vi "MainIdent RT.vi"() -> ()   [LabVIEW 2019]
doc: "The myRIO Project template acquires acceleration data from the onboard accelerometer and displays the changes of acceleration values in a waveform chart."
uses:
  <vilib>/myRIO/Common/Instrument Driver Framework/myRIO v1.0/Encoder/typedefs/Encoder Signal Mode.ctl
  <vilib>/Platform/TimedLoop/XDataNode/timing_clust.ctl
  <vilib>/Platform/TimedLoop/XDataNode/nitl_modes.ctl
  <vilib>/Platform/TimedLoop/XDataNode/wakeup.ctl
  <vilib>/myRIO/Instrument Drivers/Onboard IO/PWM/typedefs/PWM Reference.ctl
  <vilib>/myRIO/Common/Instrument Driver Framework/Utilities/typedefs/myRIO Generic Hardware Reference.ctl
  <vilib>/myRIO/Common/Instrument Driver Framework/Utilities/typedefs/Hardware Version Enum.ctl
  <vilib>/myRIO/Common/Instrument Driver Framework/Utilities/typedefs/myRIO v1.0 Reference.ctl
  <vilib>/myRIO/Common/Instrument Driver Framework/Utilities/typedefs/Generic FPGA Reference.ctl
  <vilib>/myRIO/Common/Instrument Driver Framework/myRIO v1.0/PWM/typedefs/PWM Channels Enum.ctl
  <vilib>/myRIO/Instrument Drivers/Onboard IO/PWM/typedefs/PWM Configuration.ctl
  <vilib>/userDefined/High Color/nirio_resource_hc.ctl
  <vilib>/myRIO/Common/Instrument Driver Framework/myRIO v1.0/Encoder/typedefs/Encoder Configuration v1.0.ctl
  <vilib>/myRIO/Instrument Drivers/Onboard IO/Encoder/typedefs/Encoder Reference.ctl
  <vilib>/myRIO/Common/Instrument Driver Framework/myRIO v1.0/Encoder/typedefs/Encoder Channels Enum.ctl
  <vilib>/myRIO/Common/Instrument Driver Framework/myRIO v1.0/PWM/vis/myRIO v1.1 Open PWM.vi
  <vilib>/myRIO/Common/Instrument Driver Framework/myRIO v1.0/Encoder/vis/myRIO v1.1 Open Encoder.vi
  <vilib>/myRIO/Common/Instrument Driver Framework/Utilities/vis/Validate Channels.vi
  <vilib>/myRIO/Common/Instrument Driver Framework/myRIO v1.0/PWM/vis/myRIO v1.0 Reserve PWM.vi
  <vilib>/myRIO/Instrument Drivers/Onboard IO/PWM/vis/Set Duty Cycle and Frequency.vi
  <vilib>/myRIO/Common/Instrument Driver Framework/myRIO v1.0/Encoder/vis/myRIO v1.0 Reserve Encoder.vi
  <vilib>/myRIO/Common/Instrument Driver Framework/myRIO v1.0/Encoder/vis/myRIO v1.0 Close Encoder.vi
  <vilib>/myRIO/Common/Instrument Driver Framework/myRIO v1.0/PWM/vis/myRIO v1.0 Close PWM.vi
  <vilib>/myRIO/Common/Instrument Driver Framework/myRIO v1.0/DIO/vis/myRIO v1.0 Close DIO.vi
  <vilib>/myRIO/Common/Instrument Driver Framework/myRIO v1.0/PWM/vis/myRIO v1.0 Build MUX Configuration PWM.vi
  <vilib>/myRIO/Common/Instrument Driver Framework/myRIO v1.0/Resource Manager/vis/myRIO v1.0 Reserve Channel List.vi
  <vilib>/myRIO/Common/Instrument Driver Framework/myRIO v1.0/Encoder/vis/myRIO v1.0 Build MUX Configuration Encoder.vi
  <vilib>/myRIO/Common/Instrument Driver Framework/myRIO v1.0/Encoder/vis/myRIO v1.0 Unreserve Encoder.vi
  <vilib>/myRIO/Common/Instrument Driver Framework/myRIO v1.0/PWM/vis/myRIO v1.0 Unreserve PWM.vi
  <vilib>/myRIO/Common/Instrument Driver Framework/myRIO v1.0/DIO/vis/myRIO v1.0 Unreserve DIO.vi
  <vilib>/myRIO/Common/Instrument Driver Framework/myRIO v1.0/Resource Manager/vis/myRIO v1.0 Create Configuration List.vi
  <vilib>/myRIO/Common/Instrument Driver Framework/myRIO v1.0/Resource Manager/vis/myRIO v1.0 Reserve Channel.vi
  <vilib>/myRIO/Common/Instrument Driver Framework/myRIO v1.0/Resource Manager/vis/myRIO v1.0 Unreserve Channel.vi
  <vilib>/myRIO/Common/Instrument Driver Framework/myRIO v1.0/Resource Manager/vis/myRIO v1.0 Unreserve Channel List.vi
  <vilib>/myRIO/Common/Instrument Driver Framework/myRIO v1.0/DIO/vis/myRIO v1.0 Build MUX Configuration DIO.vi
  <vilib>/myRIO/Common/Instrument Driver Framework/myRIO v1.0/Resource Manager/vis/myRIO v1.0 Build Mutex Name.vi
  <vilib>/Utility/VariantDataType/GetNumericInfo.vi
  <vilib>/Utility/error.llb/Error Cluster From Error Code.vi
  <vilib>/myRIO/Common/Instrument Driver Framework/myRIO v1.0/myRIO v1.1 Open.vi
  <vilib>/myRIO/Common/Instrument Driver Framework/Utilities/vis/IO Manager.vi
  <vilib>/myRIO/Common/Instrument Driver Framework/Utilities/vis/Configuration Manager.vi
  <vilib>/myRIO/Common/Instrument Driver Framework/myRIO v1.0/Resource Manager/vis/myRIO v1.0 Configure IO.vi
  <vilib>/myRIO/Common/Instrument Driver Framework/myRIO v1.0/myRIO v1.0 Close.vi
  <vilib>/myRIO/Common/Instrument Driver Framework/myRIO v1.0/PWM/vis/myRIO v1.0 Write PWM.vi
  <vilib>/myRIO/Common/Instrument Driver Framework/myRIO v1.0/Encoder/vis/myRIO v1.0 Configure Encoder.vi
  <vilib>/myRIO/Common/Instrument Driver Framework/myRIO v1.0/Encoder/vis/myRIO v1.0 Enable Encoder.vi
  <vilib>/myRIO/Common/Instrument Driver Framework/myRIO v1.0/Encoder/vis/myRIO v1.0 Read Encoder.vi
  <vilib>/myRIO/Common/Instrument Driver Framework/myRIO v1.0/Encoder/vis/myRIO v1.0 Shutdown Encoder.vi
  <vilib>/myRIO/Common/Instrument Driver Framework/myRIO v1.0/PWM/vis/myRIO v1.0 Shutdown PWM.vi
  <vilib>/myRIO/Common/Instrument Driver Framework/myRIO v1.0/DIO/vis/myRIO v1.0 Shutdown DIO.vi
  <vilib>/Platform/TimedLoop/XDataNode/XDataNode.xnode
  <vilib>/myRIO/Instrument Drivers/Onboard IO/PWM/vis/myRIO PWM Open.xnode
  <vilib>/myRIO/Instrument Drivers/Onboard IO/Encoder/vis/myRIO Encoder Open.xnode
  <vilib>/Platform/TimedLoop/XDataNode/XDNodeRunTimeDep.lvlib
  <vilib>/myRIO/Instrument Drivers/Onboard IO/Encoder/Encoder.lvlib
  <vilib>/myRIO/Instrument Drivers/Onboard IO/PWM/PWM.lvlib
  <vilib>/myRIO/Instrument Drivers/Onboard IO/DIO/DIO.lvlib
panel:
  in  "Reset Counter":bool
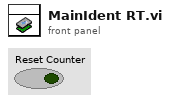
[diagram p1: front panel]
types:
  T1 = typedef "Encoder Signal Mode.ctl" = enum16{"Quadrature phase signal", "Step and direction signal"}
  T2 = typedef "PWM.lvlib/PWM Reference.ctl" = cluster{"myRIO Reference":T3, "PWM Channels Enum":T7, "PWM Configuration":T8}
  T3 = typedef "myRIO Generic Hardware Reference.ctl" = cluster{"myRIO Model":T4, "myRIO Hardware Reference":T5}
  T4 = typedef "Hardware Version Enum.ctl" = enum16{"Unknown", "myRIO-1900", "myRIO-1950", "roboRIO", "NI ELVIS RIO CM", "ELVIS III"}
  T5 = typedef "myRIO v1.0 Reference.ctl" = cluster{"Generic FPGA Reference":T6, "Allow multiple opens":bool}
  T6 = typedef "Generic FPGA Reference.ctl" = refnum<k20>
  T7 = typedef "PWM Channels Enum.ctl" = enum16{"Not Connected", "C/PWM0", "C/PWM1", "A/PWM0", "A/PWM1", "A/PWM2", "A/PWM3", "A/PWM4", "A/PWM5", "A/PWM6", "A/PWM7", "A/PWM8", "A/PWM9", "A/PWM10", "A/PWM11", "A/PWM12", "A/PWM13", "A/PWM14", "A/PWM15", "A/PWM16", "A/PWM17", "A/PWM18", "A/PWM19", "B/PWM0", "B/PWM1", "B/PWM2", "B/PWM3", "B/PWM4", "B/PWM5", "B/PWM6", "B/PWM7", "B/PWM8", "B/PWM9", "B/PWM10", "B/PWM11", "B/PWM12", "B/PWM13", "B/PWM14", "B/PWM15", "B/PWM16", "B/PWM17", "B/PWM18", "B/PWM19", "PWM/PWM0", "PWM/PWM1", "PWM/PWM2", "PWM/PWM3", "PWM/PWM4", "PWM/PWM5", "PWM/PWM6", "PWM/PWM7", "PWM/PWM8", "PWM/PWM9"}
  T8 = typedef "PWM.lvlib/PWM Configuration.ctl" = cluster{"Frequency":dbl, "Duty Cycle":dbl}
  T9 = typedef "Encoder.lvlib/Encoder Reference.ctl" = cluster{"myRIO Reference":T3, "Encoder Channels Enum":T10}
  T10 = typedef "Encoder Channels Enum.ctl" = enum16{"Not Connected", "C/ENC0", "C/ENC1", "A/ENC", "A/ENC0", "A/ENC1", "A/ENC2", "A/ENC3", "A/ENC4", "A/ENC5", "A/ENC6", "A/ENC7", "A/ENC8", "A/ENC9", "B/ENC", "B/ENC0", "B/ENC1", "B/ENC2", "B/ENC3", "B/ENC4", "B/ENC5", "B/ENC6", "B/ENC7", "B/ENC8", "B/ENC9", "DIO/ENC0", "DIO/ENC1", "DIO/ENC2", "DIO/ENC3", "DIO/ENC4"}
  T11 = typedef "DIO.lvlib/DIO Reference.ctl" = cluster{"myRIO Reference":T3, "DIO Channels List":T12}
  T12 = typedef "DIO Channels List.ctl" = T13[]
  T13 = typedef "DIO Channels Enum.ctl" = enum16{"Not Connected", "C/DIO0", "C/DIO1", "C/DIO2", "C/DIO3", "C/DIO4", "C/DIO5", "C/DIO6", "C/DIO7", "A/DIO0", "A/DIO1", "A/DIO2", "A/DIO3", "A/DIO4", "A/DIO5", "A/DIO6", "A/DIO7", "A/DIO8", "A/DIO9", "A/DIO10", "A/DIO11", "A/DIO12", "A/DIO13", "A/DIO14", "A/DIO15", "A/DIO16", "A/DIO17", "A/DIO18", "A/DIO19", "B/DIO0", "B/DIO1", "B/DIO2", "B/DIO3", "B/DIO4", "B/DIO5", "B/DIO6", "B/DIO7", "B/DIO8", "B/DIO9", "B/DIO10", "B/DIO11", "B/DIO12", "B/DIO13", "B/DIO14", "B/DIO15", "B/DIO16", "B/DIO17", "B/DIO18", "B/DIO19", "LED0", "LED1", "LED2", "LED3", "Button0", "DIO/DIO0", "DIO/DIO1", "DIO/DIO2", "DIO/DIO3", "DIO/DIO4", "DIO/DIO5", "DIO/DIO6", "DIO/DIO7", "DIO/DIO8", "DIO/DIO9", "SPI/CS0", "SPI/CS1", "SPI/CS2", "SPI/CS3", "LED RADIO (Green)", "LED RADIO (Red)", "LED COMM (Green)", "LED COMM (Red)", "LED MODE (Green)", "LED MODE (Red)"}
  T14 = typedef "XDNodeRunTimeDep.lvlib/timing_clust.ctl" = cluster{"Expected End [f-1]":u64, "Actual End [f-1]":u64, "Finished Late? [f-1]":bool, "Expected End [i-1]":u64, "Actual End [i-1]":u64, "Finished Late? [i-1]":bool, "Expected Start [i]":u64, "Actual Start [i]":u64, "Expected Start [f]":u64, "Actual Start [f]":u64, "Source Name":string, "Structure Name":string, "Period":i64, "Deadline":i64, "Offset":i64, "Start":i64, "Priority":i32, "Timeout":i32, "Mode":T15, "Wakeup Reason":T16, "Error":errorcluster, "Source Type":string, "Secondary Source Type":string, "Global End Time":u64, "Global Start Time":u64, "Frame Duration":u64, "Iteration Duration":u64, "Assigned CPU":i32, "I/O Scan Engine Mode":u32}
  T15 = typedef "XDNodeRunTimeDep.lvlib/nitl_modes.ctl" = enum32{"No Change", "Process missed periods, maintain original phase", "Discard missed periods, maintain original phase", "Process missed periods, ignore original phase", "Discard missed periods, ignore original phase"}
  T16 = typedef "XDNodeRunTimeDep.lvlib/wakeup.ctl" = enum32{"Normal", "Aborted", "Asynchronous wakeup", "Timing source error", "Timed loop error", "Timeout"}
  T17 = cluster{"setpoint (rads)":dbl, "encoder (rads)":dbl, dbl, "seconds since 1Jan1904":timestamp}
  T18 = cluster{"Double":dbl, "dbl Scaled Value":dbl, "Output":dbl, "seconds since 1Jan1904":timestamp}
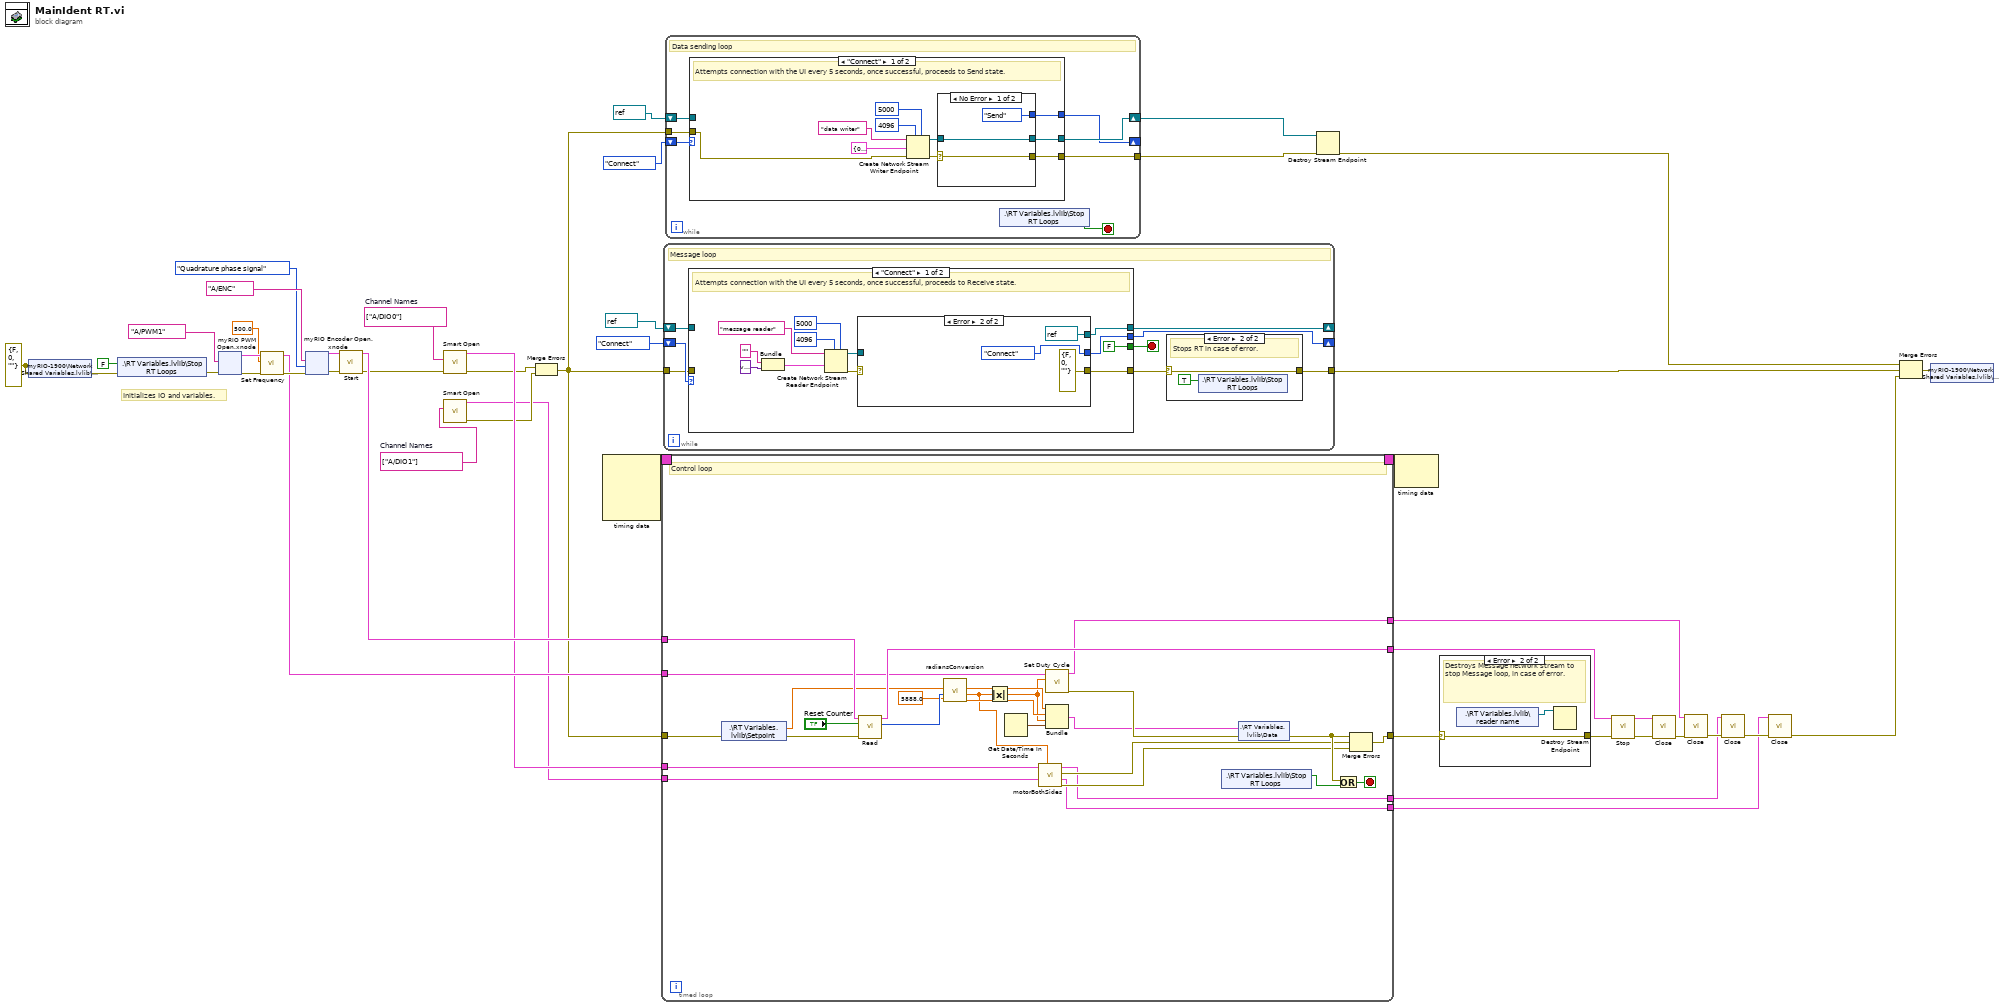
[diagram p0: block diagram]
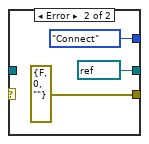
[diagram p3: hidden frame]
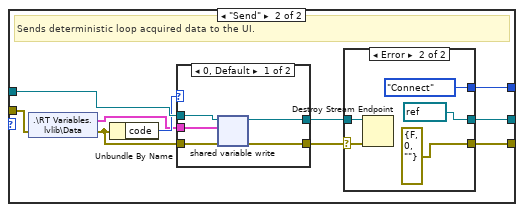
[diagram p4: hidden frame]
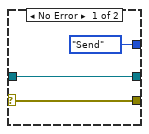
[diagram p5: hidden frame]
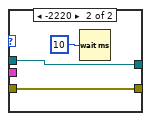
[diagram p6: hidden frame]
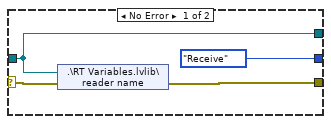
[diagram p8: hidden frame]
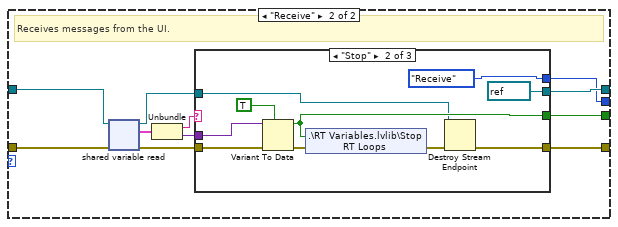
[diagram p9: hidden frame]
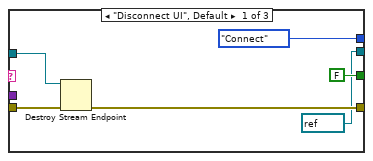
[diagram p10: hidden frame]
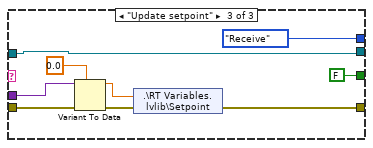
[diagram p11: hidden frame]
diagram:
  w5 = tag[] ["A/DIO1"]  # Channel Names
  w13 = tag[] ["A/DIO0"]  # Channel Names
  w33 = errorcluster {"status"=FALSE, "code"=0, "source"=""} ("error IO")
  # "Initializes IO and variables."
  n1 = shared-variable "myRIO-1900\\Network Shared Variables.lvlib\\error IO"(w33, error in=w33) -> (error out=w34:errorcluster)
  n2 = shared-variable ".\\RT Variables.lvlib\\Stop RT Loops"(FALSE ("Stop RT Loops"), error in=w34) -> (error out=w20:errorcluster)
  n3 = xnode "myRIO PWM Open.xnode"("error in (no error)"=w20, "Channel Name"=tag "A/PWM1") -> ("error out"=w22:errorcluster, "PWM Ref Out"=w21:T2)  [unwired: 1 in]
  n4 = call <vilib>:"Set Frequency.vi"("error in (no error)"=w22, "Frequency [Hz]"=500.0, "PWM Ref In"=w21) -> ("error out"=w19:errorcluster, "PWM Ref Out"=w17:T2)  [unwired: 6 in]
  n5 = xnode "myRIO Encoder Open.xnode"("error in (no error)"=w19, "Channel Name"=tag "A/ENC", "Encoder Signal Mode"=Encoder_Signal_Mode."Quadrature phase signal") -> ("error out"=w30:errorcluster, "Encoder Ref Out"=w29:T9)  [unwired: 2 in]
  n6 = call <vilib>:"Start.vi"("error in (no error)"=w30, "Encoder Ref In"=w29) -> ("error out"=w11:errorcluster, "Encoder Ref Out"=w27:T9)  [unwired: 8 in]
  n7 = call <vilib>:"Smart Open.vi"("error in (no error)"=w11, "Channel Names"=w13) -> ("error out"=w7:errorcluster, "DIO Ref Out"=w12:T11)  [unwired: 8 in]
  n8 = call <vilib>:"Smart Open.vi"("Channel Names"=w5) -> ("error out"=w6:errorcluster, "DIO Ref Out"=w4:T11)  [unwired: 9 in]
  n9 = Merge Errors(w7, w6) -> (w8:errorcluster)
  n10 = node-c288() -> (w46:T14)  [unwired: 4 in]
  n11 = timed-loop {
    timing: w46 -> [_]
    timing-out: [_] -> w45
    tunnel: w8 -> [w72]
    tunnel: [w61] -> w32
    tunnel: w27 -> [w68]
    tunnel: [w67] -> w23
    tunnel: w17 -> [w65]
    tunnel: [w64] -> w16
    tunnel: w12 -> [w49]
    tunnel: [w52] -> w9
    tunnel: w4 -> [w48]
    tunnel: [w51] -> w1
    stop <- w69 stop-if-true
    # "Control loop"
    n12 = shared-variable ".\\RT Variables.lvlib\\Setpoint"(error in=w72) -> (w58:dbl, error out=w73:errorcluster)
    n13 = call <vilib>:"Read.vi"("error in (no error)"=w73, "Reset Counter"="Reset Counter", "Encoder Ref In"=w68) -> ("Counter Value"=w59:i32, "Encoder Ref Out"=w67:T9)  [unwired: 4 in, 3 out]
    n14 = call "radiansConversion.vi"("pulses"=5888.0, "encoder"=w59, "setpoint"=w58) -> ("encoder (rads)"=w57:dbl, "error"=w50:dbl, "setpoint (rads)"=w56:dbl)  [unwired: 6 in]
    n15 = Absolute Value(x=w50) -> (abs(x)=w55:dbl)
    n16 = Get Date/Time In Seconds() -> (seconds since 1Jan1904=w71:timestamp)
    n17 = call "motorBothSides.vi"("error"=w50, "DIO Ref In 2"=w48, "DIO Ref In"=w49) -> ("error out 2"=w53:errorcluster, "DIO Ref Out 2"=w51:T11, "error out"=w54:errorcluster, "DIO Ref Out"=w52:T11)  [unwired: 5 in]
    n18 = call <vilib>:"Set Duty Cycle.vi"("Duty Cycle"=w55, "PWM Ref In"=w65) -> ("error out"=w66:errorcluster, "PWM Ref Out"=w64:T2)  [unwired: 7 in]
    n19 = Bundle("setpoint (rads)"=w56, "encoder (rads)"=w57, w55, "seconds since 1Jan1904"=w71) -> (w63:T17)  [unwired: 1 in]
    n20 = shared-variable ".\\RT Variables.lvlib\\Stop RT Loops"() -> (w70:bool)  [unwired: 1 in, 1 out]
    n21 = shared-variable ".\\RT Variables.lvlib\\Data"(w63, error in=w66) -> (error out=w60:errorcluster)
    n22 = Or(x=w60, y=w70) -> (x .or. y?=w69:bool)
    n23 = Merge Errors(w60, w54, w53) -> (w61:errorcluster)
  }
  n24 = while {
    tunnel: [w76] -> w36
    shift-right: [w82] -> _
    shift-left: refnum<k21> refnum ("reader name") -> [w80]
    shift-right: [w81] -> _
    shift-left: enum16{"Connect", "Receive"}."Connect" ("Message states") -> [w83]
    tunnel: w8 -> [w78]
    stop <- w79 stop-if-true
    # "Message loop"
    n25 = case shown="\"Connect\"" w83 {
      tunnel: [w89 w109] -> w77
      tunnel: [w88 w111] -> w82
      tunnel: [w96 w106] -> w81
      tunnel: w80 -> [_ w116]
      tunnel: w78 -> [_ w108]
      tunnel: [FALSE ("Stop RT Loops") w107] -> w79
      frame "Connect" {
        # "Attempts connection with the UI every 5 seconds, once successful, proceeds to Receive state."
        n26 = Bundle("", variant) -> (w92:cluster{string, variant})  [unwired: 1 in]
        n27 = Create Network Stream Reader Endpoint(5:5000 ("timeout in ms (-1)"), 7:4096 ("reader buffer size"), 9:w92, 11:"message reader" ("reader name")) -> (0:w91:errorcluster, 3:w87:refnum<k21>)  [unwired: 3 in]
        n28 = case shown="Error" w91 {
          selector: w91 -> [w100 _]
          tunnel: [enum16{"Connect", "Receive"}."Receive" ("Message states") enum16{"Connect", "Receive"}."Connect" ("Message states")] -> w96
          tunnel: [w99 errorcluster {"status"=FALSE, "code"=0, "source"=""} ("error IO")] -> w89
          tunnel: [w101 refnum<k21> refnum ("reader name")] -> w88
          tunnel: w87 -> [w101 _]
          frame No Error {
            n29 = shared-variable ".\\RT Variables.lvlib\\reader name"(w101, error in=w100) -> (error out=w99:errorcluster)
          }
          frame Error {
          }
        }
      }
      frame "Receive" {
        # "Receives messages from the UI."
        n30 = shared-variable-read(w116, w108) -> (w110:refnum<k21>, w112:errorcluster, w115:cluster{string, variant})  [unwired: 1 in, 1 out]
        n31 = Unbundle(w115) -> (w114:string, w113:variant)
        n32 = case shown="\"Stop\"" w114 {
          tunnel: w113 -> [_ w130 w141]
          tunnel: w112 -> [w120 w132 w140]
          tunnel: [w119 w126 w136] -> w109
          tunnel: [refnum<k21> refnum ("reader name") refnum<k21> refnum ("reader name") w135] -> w111
          tunnel: w110 -> [w118 w125 w135]
          tunnel: [FALSE ("Stop RT Loops") w129 FALSE ("Stop RT Loops")] -> w107
          tunnel: [enum16{"Connect", "Receive"}."Connect" ("Message states") enum16{"Connect", "Receive"}."Receive" ("Message states") enum16{"Connect", "Receive"}."Receive" ("Message states")] -> w106
          frame "Disconnect UI", Default {
            n33 = Destroy Stream Endpoint(8:w120, 11:w118) -> (0:w119:errorcluster)
          }
          frame "Stop" {
            n34 = Variant To Data(error in=w132, type=TRUE ("Stop RT Loops"), Variant=w130) -> (data=w129:bool, error out=w131:errorcluster)
            n35 = shared-variable ".\\RT Variables.lvlib\\Stop RT Loops"(w129, error in=w131) -> (error out=w127:errorcluster)
            n36 = Destroy Stream Endpoint(8:w127, 11:w125) -> (0:w126:errorcluster)
          }
          frame "Update setpoint" {
            n37 = Variant To Data(error in=w140, type=0.0, Variant=w141) -> (data=w138:dbl, error out=w137:errorcluster)
            n38 = shared-variable ".\\RT Variables.lvlib\\Setpoint"(w138, error in=w137) -> (error out=w136:errorcluster)
          }
        }
      }
    }
    n39 = case shown="Error" w77 {
      selector: w77 -> [w84 w85]
      tunnel: [w84 w85] -> w76
      frame No Error {
        # "No action required."
      }
      frame Error {
        # "Stops RT in case of error."
        n40 = shared-variable ".\\RT Variables.lvlib\\Stop RT Loops"(TRUE ("Stop RT Loops")) -> ()  [unwired: 1 in, 1 out]
      }
    }
  }
  n41 = while {
    shift-right: [w146] -> w39
    shift-left: refnum<k21> refnum ("writer endpoint") -> [w144]
    tunnel: [w145] -> w40
    tunnel: w8 -> [w143]
    shift-right: [w142] -> _
    shift-left: enum16{"Connect", "Send"}."Connect" ("Message states") -> [w147]
    stop <- w148 stop-if-true
    # "Data sending loop"
    n42 = case shown="\"Connect\"" w147 {
      tunnel: [w151 w167] -> w145
      tunnel: [w149 w165] -> w146
      tunnel: [w156 w168] -> w142
      tunnel: w144 -> [_ w174]
      tunnel: w143 -> [w152 w173]
      frame "Connect" {
        # "Attempts connection with the UI every 5 seconds, once successful, proceeds to Send state."
        n43 = Create Network Stream Writer Endpoint(5:5000 ("timeout in ms (-1)"), 7:4096 ("writer buffer size"), 8:w152, 9:T18 {"Double"=0.0, "dbl Scaled Value"=0.0, "Output"=0.0, "seconds since 1Jan1904"=timestamp(0 s since 1904-01-01)} ("Data"), 11:"data writer" ("writer name")) -> (0:w154:errorcluster, 3:w150:refnum<k21>)  [unwired: 2 in]
        n44 = case shown="No Error" w154 {
          selector: w154 -> [w159 _]
          tunnel: [enum16{"Connect", "Send"}."Send" ("Message states") enum16{"Connect", "Send"}."Connect" ("Message states")] -> w156
          tunnel: [w159 errorcluster {"status"=FALSE, "code"=0, "source"=""} ("error IO")] -> w151
          tunnel: w150 -> [w161 _]
          tunnel: [w161 refnum<k21> refnum ("writer endpoint")] -> w149
          frame No Error {
          }
          frame Error {
          }
        }
      }
      frame "Send" {
        # "Sends deterministic loop acquired data to the UI."
        n45 = shared-variable ".\\RT Variables.lvlib\\Data"(error in=w173) -> (w170:T18, error out=w172:errorcluster)
        n46 = Unbundle By Name(w172) -> ("code"=w171:i32)
        n47 = case shown="0, Default" w171 {
          tunnel: [w187 w189] -> w169
          tunnel: [w186 w188] -> w166
          tunnel: w174 -> [w185 w188]
          tunnel: w172 -> [w184 w189]
          tunnel: w170 -> [w183 _]
          frame 0, Default {
            n48 = shared-variable-write(w185, w184, w183) -> (w186:refnum<k21>, w187:errorcluster)  [unwired: 1 in, 1 out]
          }
          frame -2220 {
            n49 = Wait (ms)(milliseconds to wait=u32 10) -> ()  [unwired: 1 out]
          }
        }
        n50 = case shown="Error" w169 {
          selector: w169 -> [w177 w181]
          tunnel: [enum16{"Connect", "Send"}."Send" ("Message states") enum16{"Connect", "Send"}."Connect" ("Message states")] -> w168
          tunnel: [w177 errorcluster {"status"=FALSE, "code"=0, "source"=""} ("error IO")] -> w167
          tunnel: w166 -> [w175 w180]
          tunnel: [w175 refnum<k21> refnum ("writer endpoint")] -> w165
          frame No Error {
          }
          frame Error {
            n51 = Destroy Stream Endpoint(8:w181, 11:w180) -> ()  [unwired: 1 out]
          }
        }
      }
    }
    n52 = shared-variable ".\\RT Variables.lvlib\\Stop RT Loops"() -> (w148:bool)  [unwired: 1 in, 1 out]
  }
  n53 = Destroy Stream Endpoint(8:w40, 11:w39) -> (0:w37:errorcluster)
  n54 = node-c288(w45) -> ()  [unwired: 1 out]
  n55 = case shown="Error" w32 {
    selector: w32 -> [w191 w192]
    tunnel: [w191 w192] -> w24
    frame No Error {
      # "No action required."
    }
    frame Error {
      # "Destroys Message network stream to stop Message loop, in case of error."
      n56 = shared-variable ".\\RT Variables.lvlib\\reader name"() -> (w193:refnum<k21>)  [unwired: 1 in, 1 out]
      n57 = Destroy Stream Endpoint(11:w193) -> ()  [unwired: 1 in, 1 out]
    }
  }
  n58 = call <vilib>:"Stop.vi"("error in (no error)"=w24, "Encoder Ref In"=w23) -> ("error out"=w25:errorcluster, "Encoder Ref Out"=w26:T9)  [unwired: 8 in]
  n59 = call <vilib>:"Close.vi"("error in (no error)"=w25, "Encoder Ref In"=w26) -> ("error out"=w18:errorcluster)  [unwired: 9 in]
  n60 = call <vilib>:"Close.vi"("error in (no error)"=w18, "PWM Ref In"=w16) -> ("error out"=w10:errorcluster)  [unwired: 9 in]
  n61 = call <vilib>:"Close.vi"("error in (no error)"=w10, "DIO Ref In"=w9) -> ("error out"=w3:errorcluster)  [unwired: 9 in]
  n62 = call <vilib>:"Close.vi"("error in (no error)"=w3, "DIO Ref In"=w1) -> ("error out"=w2:errorcluster)  [unwired: 9 in]
  n63 = Merge Errors(w37, w36, w2) -> (w35:errorcluster)
  n64 = shared-variable "myRIO-1900\\Network Shared Variables.lvlib\\error IO"(w35) -> ()  [unwired: 1 in, 1 out]
